vi "LoadAllHardware.vi"(8 "error in (no error)":errorcluster, 11 "Microscope in":refnum<class "Microscope.lvclass">) -> (0 "error out":errorcluster, 3 "Microscope out":refnum<class "Microscope.lvclass">)   [LabVIEW 2020, in "Microscope.lvlib" / "Microscope.lvclass"]
uses:
  Microscope.lvclass
  C:/Program Files/National Instruments/LabVIEW 2020/vi.lib/ActorFramework/Actor/Actor.lvclass
  Microscope.lvclass/Microscope.ctl
  Component/Device/Device Messages/StartSequenceAcquisition Msg/StartSequenceAcquisition Msg.lvclass/StartSequenceAcquisition Msg.ctl
  <vilib>/ActorFramework/Message Enqueuer/Message Enqueuer.lvclass/Message Enqueuer.ctl
  <vilib>/ActorFramework/Message Enqueuer/Enqueue.vi
  Component/Device/Device/Device.lvclass
  Component/Device/Device Messages/StartSequenceAcquisition Msg/StartSequenceAcquisition Msg.lvclass
  C:/Program Files/National Instruments/LabVIEW 2020/vi.lib/ActorFramework/Message/Message.lvclass
  <vilib>/ActorFramework/Message Priority Queue/Priority Enqueue.vi
  <vilib>/ActorFramework/Actor/Actor.lvclass
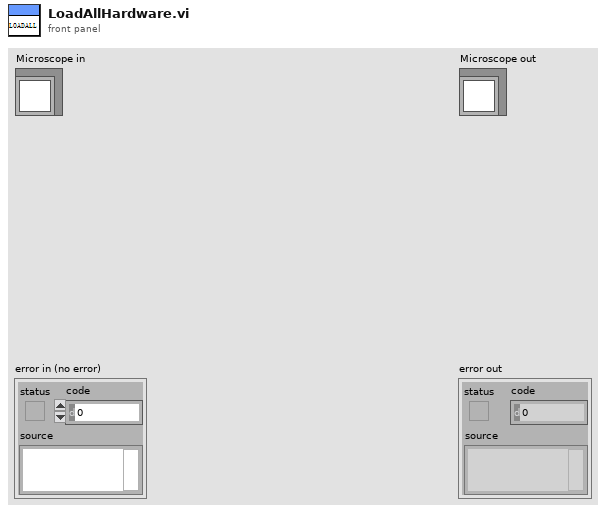
[diagram p1: front panel]
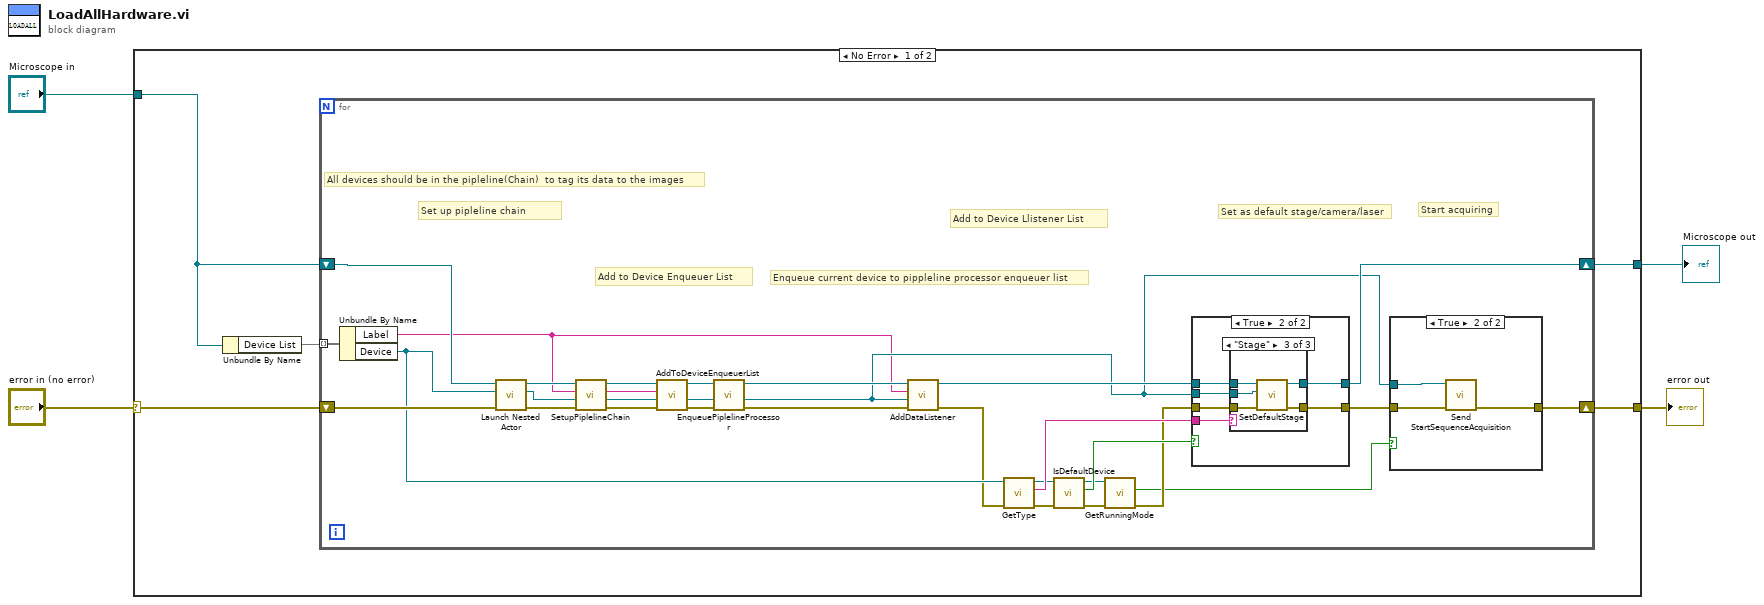
[diagram p0: block diagram]
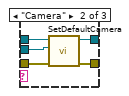
[diagram p5: hidden frame]
diagram:
  n1 = case shown="No Error" "error in (no error)" {
    selector: "error in (no error)" -> [w8 w66]
    tunnel: [w7 w66] -> w3
    tunnel: [w5 w65] -> w1
    tunnel: "Microscope in" -> [w6 w65]
    frame No Error {
      n2 = Unbundle By Name(w6) -> ("Device List"=w9:map{string, refnum<class "Device.lvclass">})
      n3 = for {
        tunnel: w9 -> [w39] mode=indexing
        shift-right: [w29] -> w7
        shift-left: w8 -> [w40]
        shift-right: [w28] -> w5
        shift-left: w6 -> [w19]
        # "Add to Device Llistener List"
        # "Start acquiring"
        # "Set as default stage/camera/laser"
        # "Enqueue current device to pippleline processor enqueuer list"
        # "Add to Device Enqueuer List"
        # "Set up pipleline chain"
        # "All devices should be in the pipleline(Chain)  to tag its data to the images"
        n4 = Unbundle By Name(w39) -> ("Label"=w10:string, "Device"=w24:refnum<class "Device.lvclass">)
        n5 = call <vilib>:"Launch Nested Actor.vi"("error in (no error)"=w40, "Nested Actor"=w24, "Caller Actor in"=w19) -> ("error out"=w27:errorcluster, "Nested Actor's Enqueuer"=w20:refnum<class "Message Enqueuer.lvclass">, "Caller Actor out"=w18:refnum<class "Microscope.lvclass">)  [unwired: 6 in]
        n6 = call-dynamic "SetupPiplelineChain.vi"("error in (no error)"=w27, "Enqueuer"=w20, "Destination"=w10, "Microscope in"=w18) -> ("error out"=w23:errorcluster, "Enqueuer dup"=w16:refnum<class "Message Enqueuer.lvclass">, "Destination dup"=w17:string, "Microscope out"=w22:refnum<class "Microscope.lvclass">)  [unwired: 4 in]
        n7 = call-dynamic "AddToDeviceEnqueuerList.vi"("error in (no error)"=w23, "DeviceEnqueuer"=w16, "Label"=w17, "Microscope in"=w22) -> ("error out"=w26:errorcluster, "DeviceEnqueuer dup"=w15:refnum<class "Message Enqueuer.lvclass">, "Microscope out"=w21:refnum<class "Microscope.lvclass">)  [unwired: 4 in, 1 out]
        n8 = call-dynamic "EnqueuePiplelineProcessor.vi"("error in (no error)"=w26, "Enqueuer"=w15, "Microscope in"=w21) -> ("error out"=w25:errorcluster, "Enqueuer out"=w11:refnum<class "Message Enqueuer.lvclass">, "Microscope out"=w13:refnum<class "Microscope.lvclass">)  [unwired: 6 in]
        n9 = call-dynamic "AddDataListener.vi"("error in (no error)"=w25, "Listener In"=w11, "Label"=w10, "GRMActor in"=w13) -> ("error out"=w14:errorcluster, "GRMActor out"=w12:refnum<class "Microscope.lvclass">)  [unwired: 6 in]
        n10 = call-dynamic "GetType.vi"("error in (no error)"=w14, "GRMActor in"=w24) -> ("error out"=w37:errorcluster, "Type"=w36:string, "GRMActor out"=w34:refnum<class "Device.lvclass">)  [unwired: 7 in]
        n11 = call-dynamic "IsDefaultDevice.vi"("error in (no error)"=w37, "Device in"=w34) -> ("error out"=w35:errorcluster, "DefaultDevice?"=w33:bool, "Device out"=w31:refnum<class "Device.lvclass">)  [unwired: 7 in]
        n12 = call-dynamic "GetRunningMode.vi"("error in (no error)"=w35, "Device in"=w31) -> ("error out"=w32:errorcluster, "RunAfterLoaded?"=w30:bool)  [unwired: 7 in, 1 out]
        n13 = case shown="True" w33 {
          tunnel: w32 -> [w45 w50]
          tunnel: w12 -> [w46 w51]
          tunnel: [w46 w48] -> w28
          tunnel: [w45 w49] -> w38
          tunnel: w36 -> [_ w52]
          tunnel: w11 -> [_ w47]
          frame False {
          }
          frame True {
            n14 = case shown="\"Stage\"" w52 {
              tunnel: w51 -> [w54 w57 w62]
              tunnel: w50 -> [w53 w59 w64]
              tunnel: [w53 w58 w63] -> w49
              tunnel: [w54 w56 w61] -> w48
              tunnel: w47 -> [_ w55 w60]
              frame Default {
              }
              frame "Camera" {
                n15 = call-dynamic "SetDefaultCamera.vi"("error in (no error)"=w59, "DefaultCameraEnqueuer"=w55, "Microscope in"=w57) -> ("error out"=w58:errorcluster, "Microscope out"=w56:refnum<class "Microscope.lvclass">)  [unwired: 7 in]
              }
              frame "Stage" {
                n16 = call-dynamic "SetDefaultStage.vi"("error in (no error)"=w64, "DefaultStageEnqueuer"=w60, "Microscope in"=w62) -> ("error out"=w63:errorcluster, "Microscope out"=w61:refnum<class "Microscope.lvclass">)  [unwired: 7 in]
              }
            }
          }
        }
        n17 = case shown="True" w30 {
          tunnel: w38 -> [w41 w44]
          tunnel: [w41 w43] -> w29
          tunnel: w11 -> [_ w42]
          frame False {
          }
          frame True {
            n18 = call "Send StartSequenceAcquisition.vi"("error in (no error)"=w44, "Message Enqueuer"=w42) -> ("error out"=w43:errorcluster)  [unwired: 8 in, 1 out]
          }
        }
      }
    }
    frame Error {
    }
  }
  "error out" <- w3
  "Microscope out" <- w1
